vi "Terminal-PressureSystem-Getter20150815.vi"(8 "error in (no error)":errorcluster caption="错误输入（无错误）", 11 "read operation timeout (ms)":i32=5000 caption="读操作超时（5000毫秒）") -> (0 "error out":errorcluster caption="错误输出", 2 "时间标识":timestamp, 3 "设备信息":T1)   [LabVIEW 2014]
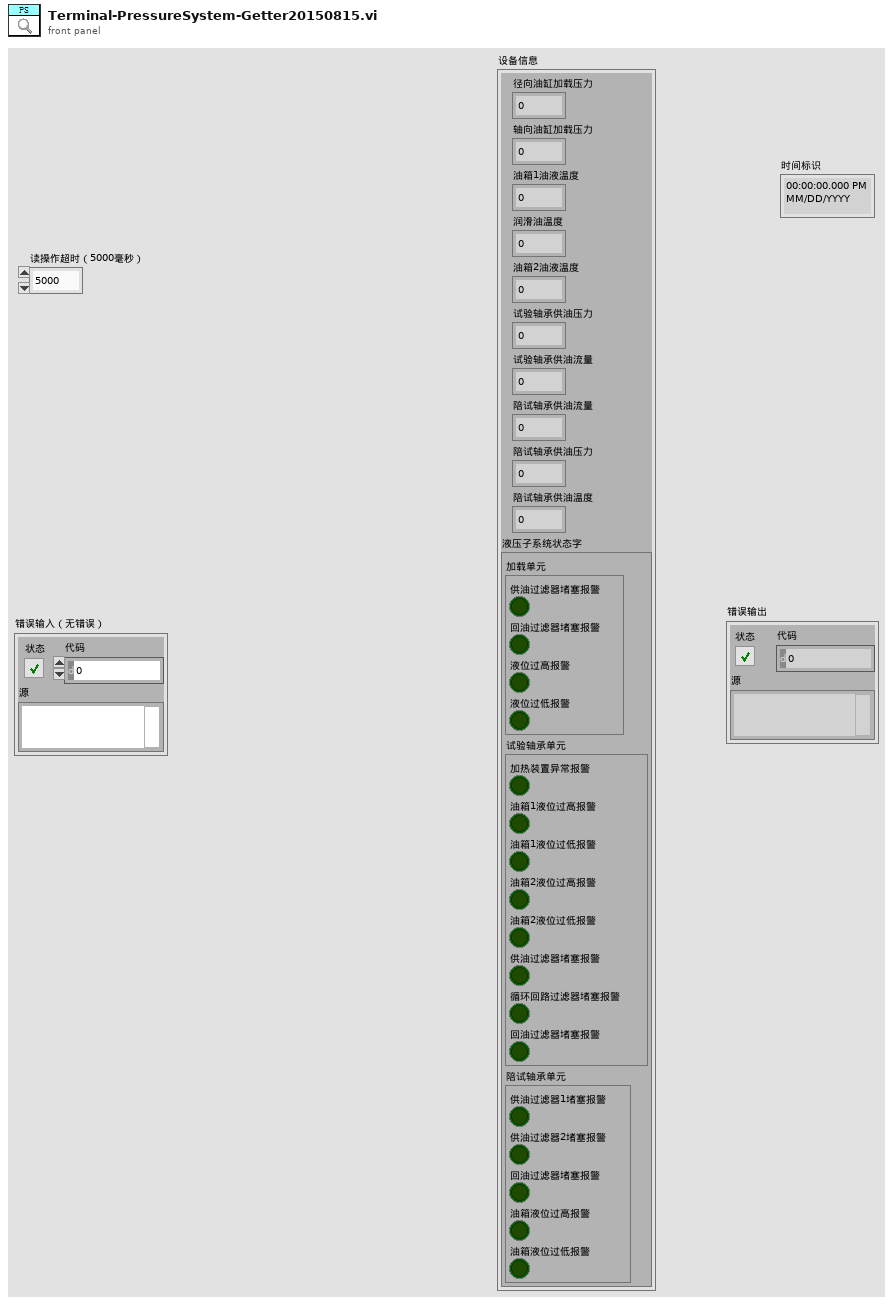
[diagram p1: front panel]
types:
  T1 = cluster{"径向油缸加载压力":u16, "轴向油缸加载压力":u16, "油箱1油液温度":u16, "润滑油温度":u16, "油箱2油液温度":u16, "试验轴承供油压力":u16, "试验轴承供油流量":u16, "陪试轴承供油流量":u16, "陪试轴承供油压力":u16, "陪试轴承供油温度":u16, "液压子系统状态字":cluster{"加载单元":cluster{"供油过滤器堵塞报警":bool, "回油过滤器堵塞报警":bool, "液位过高报警":bool, "液位过低报警":bool}, "试验轴承单元":cluster{"加热装置异常报警":bool, "油箱1液位过高报警":bool, "油箱1液位过低报警":bool, "油箱2液位过高报警":bool, "油箱2液位过低报警":bool, "供油过滤器堵塞报警":bool, "循环回路过滤器堵塞报警":bool, "回油过滤器堵塞报警":bool}, "陪试轴承单元":cluster{"供油过滤器1堵塞报警":bool, "供油过滤器2堵塞报警":bool, "回油过滤器堵塞报警":bool, "油箱液位过高报警":bool, "油箱液位过低报警":bool}}}
  T2 = cluster{"加载单元":cluster{"供油过滤器堵塞报警":bool, "回油过滤器堵塞报警":bool, "液位过高报警":bool, "液位过低报警":bool}, "试验轴承单元":cluster{"加热装置异常报警":bool, "油箱1液位过高报警":bool, "油箱1液位过低报警":bool, "油箱2液位过高报警":bool, "油箱2液位过低报警":bool, "供油过滤器堵塞报警":bool, "循环回路过滤器堵塞报警":bool, "回油过滤器堵塞报警":bool}, "陪试轴承单元":cluster{"供油过滤器1堵塞报警":bool, "供油过滤器2堵塞报警":bool, "回油过滤器堵塞报警":bool, "油箱液位过高报警":bool, "油箱液位过低报警":bool}}
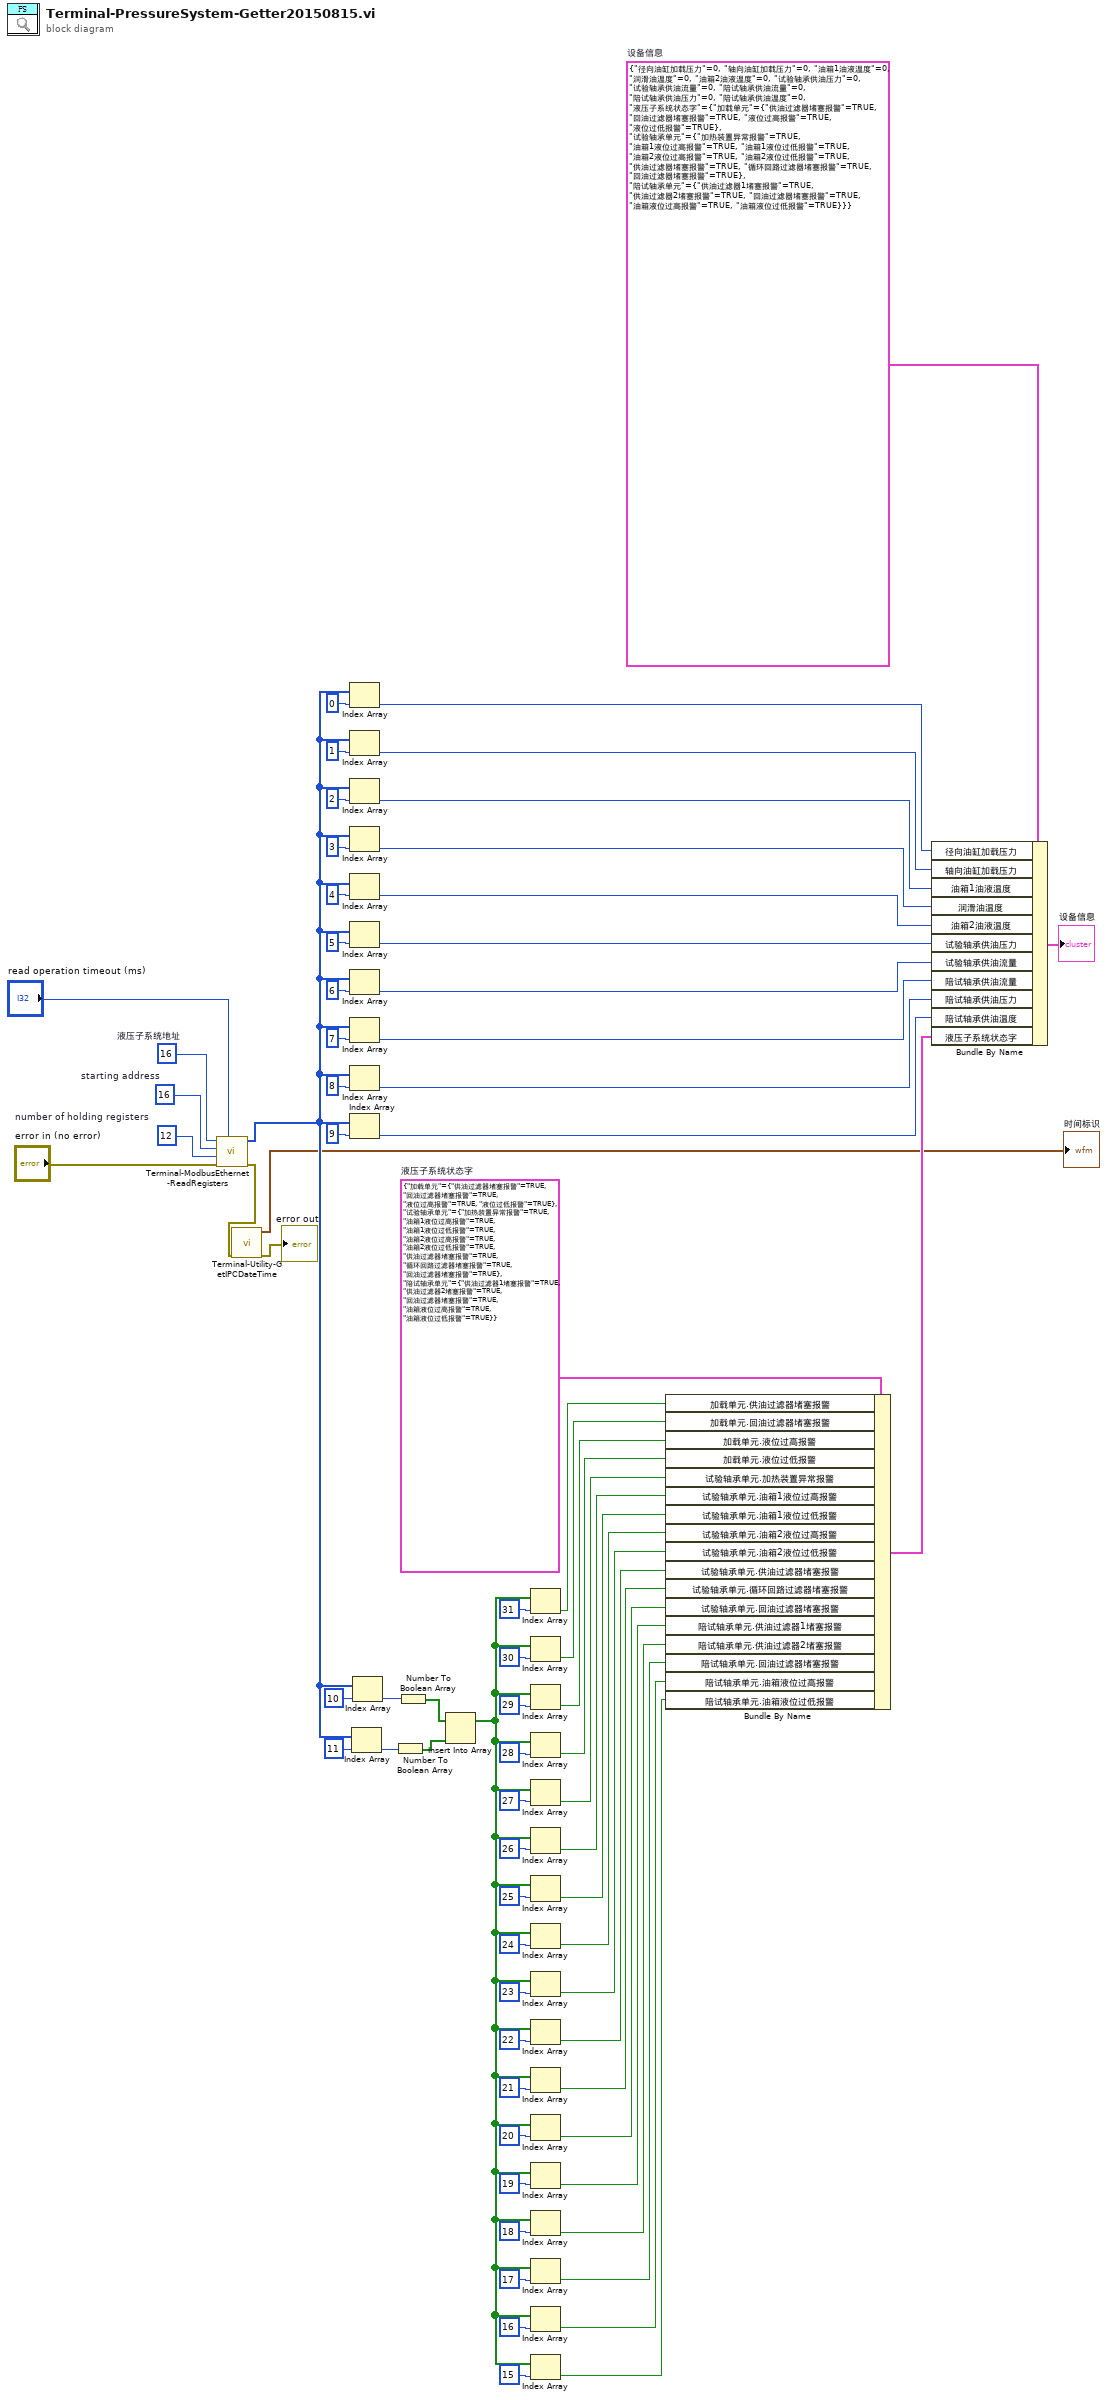
[diagram p0: block diagram]
diagram:
  w23 = T2 {"加载单元"={"供油过滤器堵塞报警"=TRUE, "回油过滤器堵塞报警"=TRUE, "液位过高报警"=TRUE, "液位过低报警"=TRUE}, "试验轴承单元"={"加热装置异常报警"=TRUE, "油箱1液位过高报警"=TRUE, "油箱1液位过低报警"=TRUE, "油箱2液位过高报警"=TRUE, "油箱2液位过低报警"=TRUE, "供油过滤器堵塞报警"=TRUE, "循环回路过滤器堵塞报警"=TRUE, "回油过滤器堵塞报警"=TRUE}, "陪试轴承单元"={"供油过滤器1堵塞报警"=TRUE, "供油过滤器2堵塞报警"=TRUE, "回油过滤器堵塞报警"=TRUE, "油箱液位过高报警"=TRUE, "油箱液位过低报警"=TRUE}}  # 液压子系统状态字
  w69 = T1 {"径向油缸加载压力"=0, "轴向油缸加载压力"=0, "油箱1油液温度"=0, "润滑油温度"=0, "油箱2油液温度"=0, "试验轴承供油压力"=0, "试验轴承供油流量"=0, "陪试轴承供油流量"=0, "陪试轴承供油压力"=0, "陪试轴承供油温度"=0, "液压子系统状态字"={"加载单元"={"供油过滤器堵塞报警"=TRUE, "回油过滤器堵塞报警"=TRUE, "液位过高报警"=TRUE, "液位过低报警"=TRUE}, "试验轴承单元"={"加热装置异常报警"=TRUE, "油箱1液位过高报警"=TRUE, "油箱1液位过低报警"=TRUE, "油箱2液位过高报警"=TRUE, "油箱2液位过低报警"=TRUE, "供油过滤器堵塞报警"=TRUE, "循环回路过滤器堵塞报警"=TRUE, "回油过滤器堵塞报警"=TRUE}, "陪试轴承单元"={"供油过滤器1堵塞报警"=TRUE, "供油过滤器2堵塞报警"=TRUE, "回油过滤器堵塞报警"=TRUE, "油箱液位过高报警"=TRUE, "油箱液位过低报警"=TRUE}}}  # 设备信息
  w72 = u16 12  # number of holding registers
  w73 = u16 16  # starting address
  w74 = u8 16  # 液压子系统地址
  n1 = call "Terminal-ModbusEthernet-ReadRegisters.vi"("read operation timeout (ms)"="read operation timeout (ms)", "error in"="error in (no error)", "number of holding registers"=w72, "starting address"=w73, "unit ID"=w74) -> ("error out"=w3:errorcluster, "register values"=w10:u16[])  [unwired: 5 in]
  n2 = call "Terminal-Utility-GetIPCDateTime.vi"("error in (no error)"=w3) -> ("error out"=→"error out":errorcluster, "时间标识"=→"时间标识":timestamp)  [unwired: 9 in]
  n3 = Index Array(array=w10, index=0 ("索引")) -> (element=w67:u16)
  n4 = Index Array(array=w10, index=1 ("索引")) -> (element=w63:u16)
  n5 = Index Array(array=w10, index=2 ("索引")) -> (element=w62:u16)
  n6 = Index Array(array=w10, index=3 ("索引")) -> (element=w61:u16)
  n7 = Index Array(array=w10, index=4 ("索引")) -> (element=w46:u16)
  n8 = Index Array(array=w10, index=5 ("索引")) -> (element=w45:u16)
  n9 = Index Array(array=w10, index=6 ("索引")) -> (element=w44:u16)
  n10 = Index Array(array=w10, index=7 ("索引")) -> (element=w43:u16)
  n11 = Index Array(array=w10, index=8 ("索引")) -> (element=w42:u16)
  n12 = Index Array(array=w10, index=9 ("索引")) -> (element=w41:u16)
  n13 = Index Array(array=w10, index=11 ("索引")) -> (element=w7:u16)
  n14 = Index Array(array=w10, index=10 ("索引")) -> (element=w8:u16)
  n15 = Number To Boolean Array(number=w7) -> (Boolean array=w5:bool[])
  n16 = Number To Boolean Array(number=w8) -> (Boolean array=w6:bool[])
  n17 = Insert Into Array(array=w6, new element=w5) -> (w4:bool[])  [unwired: 1 in]
  n18 = Index Array(array=w4, index=31 ("索引")) -> (element=w56:bool)
  n19 = Index Array(array=w4, index=30 ("索引")) -> (element=w55:bool)
  n20 = Index Array(array=w4, index=29 ("索引")) -> (element=w54:bool)
  n21 = Index Array(array=w4, index=28 ("索引")) -> (element=w53:bool)
  n22 = Index Array(array=w4, index=27 ("索引")) -> (element=w33:bool)
  n23 = Index Array(array=w4, index=26 ("索引")) -> (element=w32:bool)
  n24 = Index Array(array=w4, index=25 ("索引")) -> (element=w31:bool)
  n25 = Index Array(array=w4, index=24 ("索引")) -> (element=w30:bool)
  n26 = Index Array(array=w4, index=23 ("索引")) -> (element=w29:bool)
  n27 = Index Array(array=w4, index=22 ("索引")) -> (element=w28:bool)
  n28 = Index Array(array=w4, index=21 ("索引")) -> (element=w25:bool)
  n29 = Index Array(array=w4, index=20 ("索引")) -> (element=w24:bool)
  n30 = Index Array(array=w4, index=19 ("索引")) -> (element=w16:bool)
  n31 = Index Array(array=w4, index=18 ("索引")) -> (element=w15:bool)
  n32 = Index Array(array=w4, index=17 ("索引")) -> (element=w14:bool)
  n33 = Index Array(array=w4, index=16 ("索引")) -> (element=w13:bool)
  n34 = Index Array(array=w4, index=15 ("索引")) -> (element=w12:bool)
  n35 = Bundle By Name(cluster=w23, "加载单元.供油过滤器堵塞报警"=w56, "加载单元.回油过滤器堵塞报警"=w55, "加载单元.液位过高报警"=w54, "加载单元.液位过低报警"=w53, "试验轴承单元.加热装置异常报警"=w33, "试验轴承单元.油箱1液位过高报警"=w32, "试验轴承单元.油箱1液位过低报警"=w31, "试验轴承单元.油箱2液位过高报警"=w30, "试验轴承单元.油箱2液位过低报警"=w29, "试验轴承单元.供油过滤器堵塞报警"=w28, "试验轴承单元.循环回路过滤器堵塞报警"=w25, "试验轴承单元.回油过滤器堵塞报警"=w24, "陪试轴承单元.供油过滤器1堵塞报警"=w16, "陪试轴承单元.供油过滤器2堵塞报警"=w15, "陪试轴承单元.回油过滤器堵塞报警"=w14, "陪试轴承单元.油箱液位过高报警"=w13, "陪试轴承单元.油箱液位过低报警"=w12) -> (w40:T2)
  n36 = Bundle By Name(cluster=w69, "径向油缸加载压力"=w67, "轴向油缸加载压力"=w63, "油箱1油液温度"=w62, "润滑油温度"=w61, "油箱2油液温度"=w46, "试验轴承供油压力"=w45, "试验轴承供油流量"=w44, "陪试轴承供油流量"=w43, "陪试轴承供油压力"=w42, "陪试轴承供油温度"=w41, "液压子系统状态字"=w40) -> (→"设备信息":T1)
